vi "Configure Sequence Trig Find.vi"(0 "VISA resource name":refnum<visa-resource-name>, 1 "Find (0: Pattern 1 Entered)":u16(ring) items=["Pattern 1 Entered", "Pattern 1 Exited", "Edge 1", "Pattern 1 and Edge 1"], 11 "error in (no error)":errorcluster) -> (4 "VISA resource name out":refnum<visa-resource-name>, 15 "error out":errorcluster)   [LabVIEW 2017, in "Agilent 6000 Series.lvlib"]
doc: "This VI configures the Sequence trigger. You specify the trigger find with the Find parameter.\n\n<B>NOTE:</B>\n\nThis VI is only valid for 6000 Series models. An error will be thrown if this VI is run with 5000 Series scopes."
uses:
  <instrlib>/Agilent 6000 Series/Agilent 6000 Series.lvlib
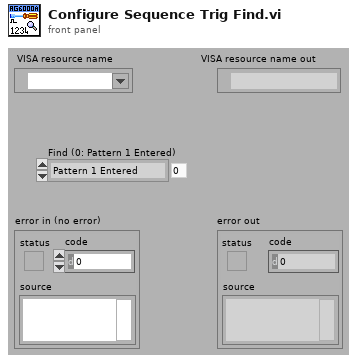
[diagram p1: front panel]
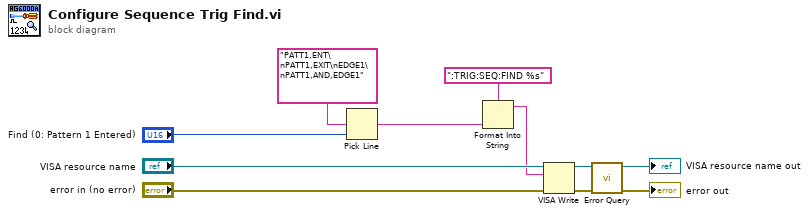
[diagram p0: block diagram]
diagram:
  n1 = Pick Line(multi-line string="PATT1,ENT\nPATT1,EXIT\nEDGE1\nPATT1,AND,EDGE1", line index="Find (0: Pattern 1 Entered)") -> (output string=w2:string)  [unwired: 1 in]
  n2 = Format Into String(format string=":TRIG:SEQ:FIND %s" ("Source Command"), w2) -> (resulting string=w4:string)  [unwired: 2 in, 1 out]
  n3 = VISA Write(VISA resource name="VISA resource name", write buffer=w4, error in (no error)="error in (no error)") -> (VISA resource name out=w7:refnum<visa-resource-name>, error out=w6:errorcluster)  [unwired: 1 out]
  n4 = call <instrlib>:"Error Query.vi"("error in (no error)"=w6, "VISA resource name"=w7) -> ("error out"=→"error out":errorcluster, "VISA resource name out"=→"VISA resource name out":refnum<visa-resource-name>)  [unwired: 6 in, 2 out]
